vi "_findOpenStorage.vi"(4 "error in (no error)":errorcluster, 6 "Storage type":string="USI", 7 "Storage location":path) -> (0 "error out":errorcluster, 3 "storage refnum":refnum<k20>)   [LabVIEW 2017]
uses:
  <resource>/objmgr/Storage.rc
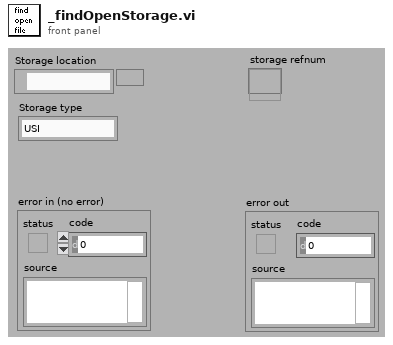
[diagram p1: front panel]
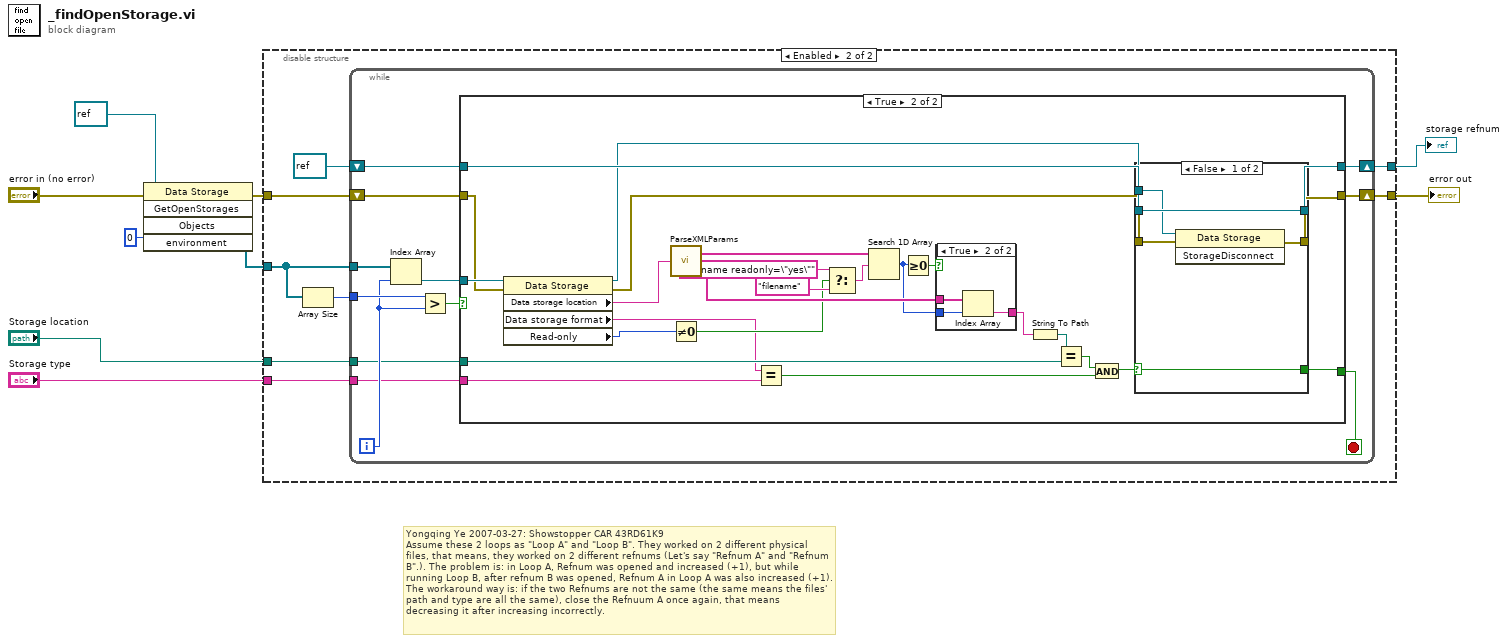
[diagram p0: block diagram]
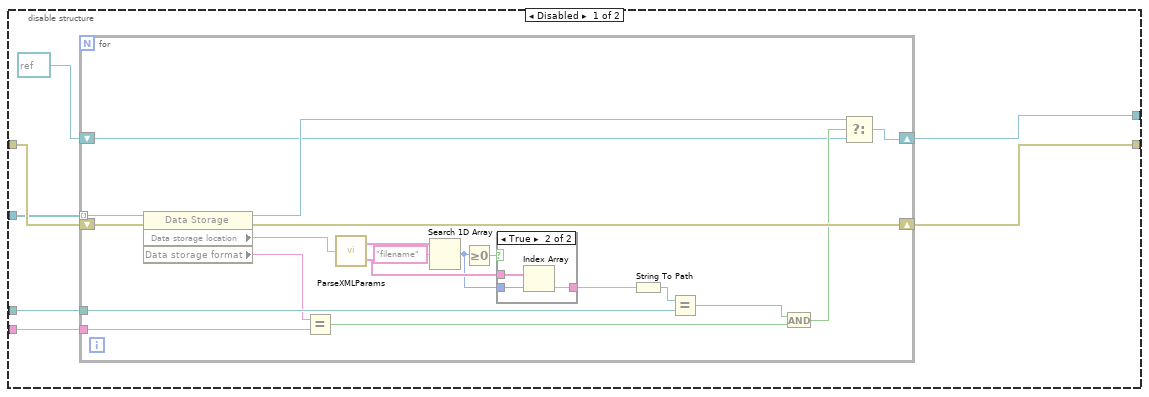
[diagram p2: hidden frame]
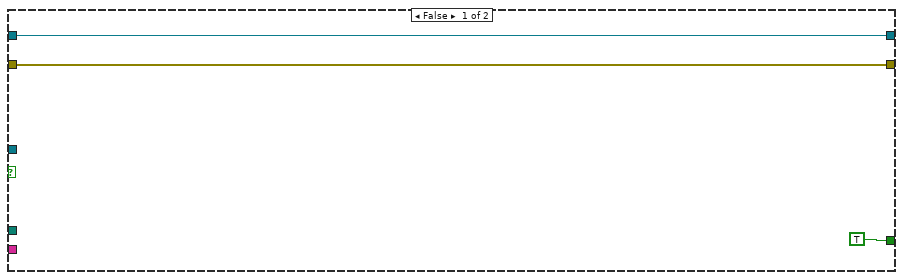
[diagram p4: hidden frame]
diagram:
  # "Yongqing Ye 2007-03-27: Showstopper CAR 43RD61K9\nAssume these 2 loops as \"Loop A\" and \"Loop B\". They worked on 2 different physical files, that means, they worked on 2 different refnums (Let's say \"Refnum A\" and \"Refnum B\".). The problem is: in Loop A, Refnum was opened and increased (+1), but while running Loop B, after refnum B was opened, Refnum A in Loop A was also increased (+1). The workaround way is: if the two Refnums are not the same (the same means the files' path and type are all the same), close the Refnuum A once again, that means decreasing it after increasing incorrectly."
  n1 = invoke class="Data Storage" method="GetOpenStorages"(reference=refnum<k20> refnum, error in="error in (no error)", "environment"=0) -> (error out=w4:errorcluster, "Objects"=w3:refnum<k20>[])  [unwired: 2 in, 3 out]
  n2 = disable-structure shown="Enabled" {
    disable-tunnel: [w16 w40] -> w9
    disable-tunnel: "Storage type" -> [w15 w42]
    disable-tunnel: "Storage location" -> [w14 w43]
    disable-tunnel: [w13 w41] -> w5
    disable-tunnel: w4 -> [w12 w44]
    disable-tunnel: w3 -> [w11 w46]
    frame Disabled {
      n3 = for {
        tunnel: w11 -> [w36] mode=indexing
        shift-right: [w34] -> w16
        shift-left: w12 -> [w35]
        tunnel: w14 -> [w25]
        tunnel: w15 -> [w24]
        shift-right: [w17] -> w13
        shift-left: refnum<k20> refnum ("reference") -> [w18]
        n4 = property class="Data Storage"(reference=w36, error in=w35) -> (reference out=w19:refnum<k20>, error out=w34:errorcluster, "Data storage location"=w28:string, "Data storage format"=w23:string)
        n5 = Equal?(x=w23, y=w24) -> (x = y?=w22:bool)
        n6 = call <vilib>:"ParseXMLParams.vi"("Parameter String"=w28) -> ("Names"=w33:string[], "Values"=w30:string[])
        n7 = Search 1D Array(1D array=w33, element="filename") -> (index of element=w29:i32)  [unwired: 1 in]
        n8 = Greater Or Equal To 0?(x=w29) -> (x >= 0?=w31:bool)
        n9 = case shown="True" w31 {
          tunnel: w30 -> [_ w39]
          tunnel: w29 -> [_ w38]
          tunnel: [_ w37] -> w27
          frame False {
          }
          frame True {
            n10 = Index Array(array=w39, index=w38) -> (element=w37:string)
          }
        }
        n11 = String To Path(string=w27) -> (path=w26:path)
        n12 = Equal?(x=w26, y=w25) -> (x = y?=w21:bool)
        n13 = And(x=w21, y=w22) -> (x .and. y?=w20:bool)
        n14 = Select(t=w19, s=w20, f=w18) -> (s? t:f=w17:refnum<k20>)
      }
    }
    frame Enabled {
      n15 = Array Size(array=w46) -> (size(s)=w47:i32)
      n16 = while {
        tunnel: w47 -> [w59]
        tunnel: w46 -> [w57]
        shift-right: [w48] -> w41
        shift-left: refnum<k20> refnum ("reference") -> [w54]
        tunnel: w43 -> [w52]
        tunnel: w42 -> [w51]
        shift-right: [w49] -> w40
        shift-left: w44 -> [w53]
        i -> [w56]
        stop <- w50 stop-if-true
        n17 = Index Array(array=w57, index=w56) -> (element=w55:refnum<k20>)
        n18 = Greater?(x=w59, y=w56) -> (0:w58:bool)
        n19 = case shown="True" w58 {
          tunnel: w55 -> [_ w69]
          tunnel: w54 -> [w60 w82]
          tunnel: w53 -> [w61 w68]
          tunnel: w52 -> [_ w86]
          tunnel: w51 -> [_ w85]
          tunnel: [TRUE w80] -> w50
          tunnel: [w61 w81] -> w49
          tunnel: [w60 w83] -> w48
          frame False {
          }
          frame True {
            n20 = property class="Data Storage"(reference=w69, error in=w68) -> (reference out=w67:refnum<k20>, error out=w66:errorcluster, "Data storage location"=w65:string, "Data storage format"=w63:string, "Read-only"=w64:i32)
            n21 = call <vilib>:"ParseXMLParams.vi"("Parameter String"=w65) -> ("Names"=w79:string[], "Values"=w77:string[])
            n22 = Not Equal To 0?(x=w64) -> (x != 0?=w72:bool)
            n23 = Equal?(x=w63, y=w85) -> (x = y?=w88:bool)
            n24 = Select(t="filename readonly=\"yes\"", s=w72, f="filename" ("element")) -> (s? t:f=w73:string)
            n25 = Search 1D Array(1D array=w79, element=w73) -> (index of element=w76:i32)  [unwired: 1 out]
            n26 = Greater Or Equal To 0?(x=w76) -> (x >= 0?=w78:bool)
            n27 = case shown="True" w78 {
              tunnel: w77 -> [_ w91]
              tunnel: w76 -> [_ w90]
              tunnel: [_ w89] -> w71
              frame False {
              }
              frame True {
                n28 = Index Array(array=w91, index=w90) -> (element=w89:string)
              }
            }
            n29 = String To Path(string=w71) -> (path=w70:path)
            n30 = Equal?(x=w70, y=w86) -> (x = y?=w87:bool)
            n31 = And(x=w87, y=w88) -> (x .and. y?=w84:bool)
            n32 = case shown="False" w84 {
              selector: w84 -> [w95 w98]
              tunnel: w67 -> [w92 w99]
              tunnel: [w96 w99] -> w83
              tunnel: w66 -> [w94 w97]
              tunnel: w82 -> [w96 _]
              tunnel: [w93 w97] -> w81
              tunnel: [w95 w98] -> w80
              frame False {
                n33 = invoke class="Data Storage" method="StorageDisconnect"(reference=w92, error in=w94) -> (error out=w93:errorcluster)  [unwired: 1 in, 2 out]
              }
              frame True {
              }
            }
          }
        }
      }
    }
  }
  "error out" <- w9
  "storage refnum" <- w5
